vi "Erase Curve.vi"(7 "Erase Curve (T: Yes)":bool=TRUE, 8 "error in (no error)":errorcluster, 10 "Curve to Erase (21)":dbl=21.0, 11 "VISA resource name":refnum<visa-resource-name>) -> (0 "error out":errorcluster, 3 "VISA resource name out":refnum<visa-resource-name>)   [LabVIEW 2019, in "Lake Shore 335.lvlib"]
doc: "Erases a user curve. Erasing the curve sets all identification parameters to default and blanks all breakpoint values."
uses:
  Lake Shore 335.lvlib
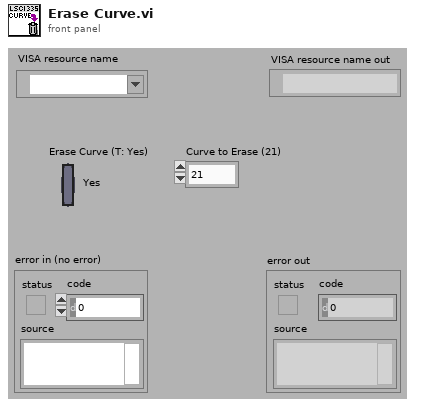
[diagram p1: front panel]
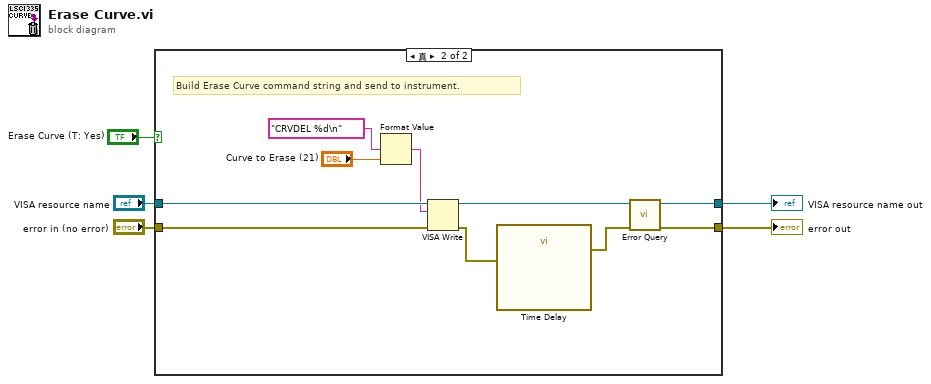
[diagram p0: block diagram]
diagram:
  n1 = case shown="真" "Erase Curve (T: Yes)" {
    tunnel: "VISA resource name" -> [w7 w17]
    tunnel: "error in (no error)" -> [w6 w16]
    tunnel: [w7 w14] -> w3
    tunnel: [w6 w13] -> w2
    frame False {
      # "Do not erase curve"
    }
    frame True {
      # "Build Erase Curve command string and send to instrument."
      n2 = Format Value(format string="CRVDEL %d\n", value (0)="Curve to Erase (21)") -> (output string=w11:string)  [unwired: 1 in]
      n3 = VISA Write(VISA resource name=w17, write buffer=w11, error in (no error)=w16) -> (VISA resource name out=w15:refnum<visa-resource-name>, error out=w9:errorcluster)  [unwired: 1 out]
      n4 = call "Time Delay"("error in (no error)"=w9) -> ("error out"=w8:errorcluster)  [unwired: 10 in]
      n5 = call "Error Query.vi"("error in (no error)"=w8, "VISA resource name"=w15) -> ("error out"=w13:errorcluster, "VISA resource name out"=w14:refnum<visa-resource-name>)  [unwired: 7 in, 1 out]
    }
  }
  "VISA resource name out" <- w3
  "error out" <- w2
